vi "Set_Items.MulticolumnListbox.vi"(8 "error in (no error)":errorcluster, 9 "Strings Array In (2D)":string[][](array[string]), 10 "Listbox Name In":string, 11 "Data Value Reference in":T1) -> (0 "error out":errorcluster, 2 "reference out":refnum<vi>, 3 "Data Value Reference in 2":T1)   [LabVIEW 2020, in "CtlReferences.lvlib" / "CtlReferences.lvclass"]
uses:
  CtlReferences.lvclass
  GetControlRef/GetControl_MultiColumnListBox.vi
  TypeDefs/CtlLookup.ctl
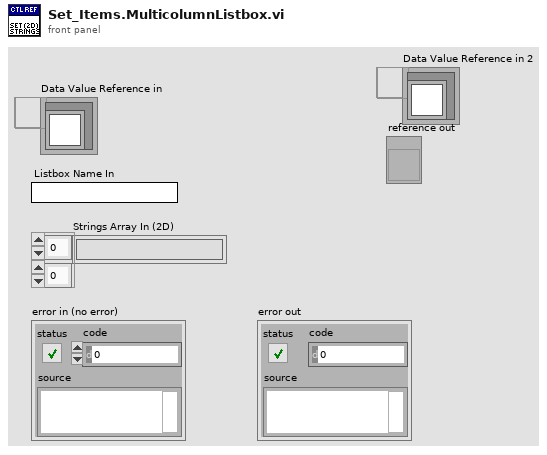
[diagram p1: front panel]
types:
  T1 = typedef "CtlReferences.lvlib/CtlReferences.lvclass/CtlLookup.ctl" = refnum<data-value>
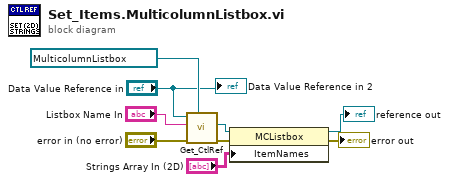
[diagram p0: block diagram]
diagram:
  n1 = call-poly "Get_CtlRef.vi"("Control Class"=refnum<vi> refnum, "error in (no error)"="error in (no error)", "Control Label"="Listbox Name In", "CtlLookup In"="Data Value Reference in") -> ("error out"=w5:errorcluster, "Reference Out"=w6:refnum<vi>)  [unwired: 5 in, 1 out]
  n2 = property class="MCListbox"(reference=w6, error in=w5, "ItemNames"="Strings Array In (2D)") -> (reference out=→"reference out":refnum<vi>, error out=→"error out":errorcluster)
  "Data Value Reference in 2" <- "Data Value Reference in"
